vi "Test Manipulator API.vi"() -> ()   [LabVIEW 2020]
doc: "Manipulator API Tester."
uses:
  Settings/Named Position.ctl
  Manipulator.lvlib
panel:
  in  "Get Module Data":bool
  in  "Position Name":string
  out "Selected Target Position":string
  in  "Named Positions":i32(listbox)
  in  "Delete Named Position":bool
  in  "Add Named Position":bool
  in  "Move to Named Position":bool
  out "Axis Indicator":bool[](array[boolean])
  out "Speed (g)":dbl[](array[numeric])
  out "Pos (g)":dbl[](array[numeric])
  in  "Speed (s)":dbl[](array[numeric])
  in  "Pos (s)":dbl[](array[numeric])
  in  "Axis":i32
  in  "Move Axis with Speed":bool
  in  "Get Status":bool
  in  "Move Axis":bool
  in  "Get Position and Speed":bool
  out "Num Axes":i32
  in  "Get Num Axes":bool
  in  "Show Block Diagram":bool
  in  "Stop Module":bool
  in  "Start Module":bool
  in  "Hide Module Panel":bool
  in  "Show Module Panel":bool
  out "Status":string
  out "Module Running?":bool
  # "This VI tests the API for the Module."
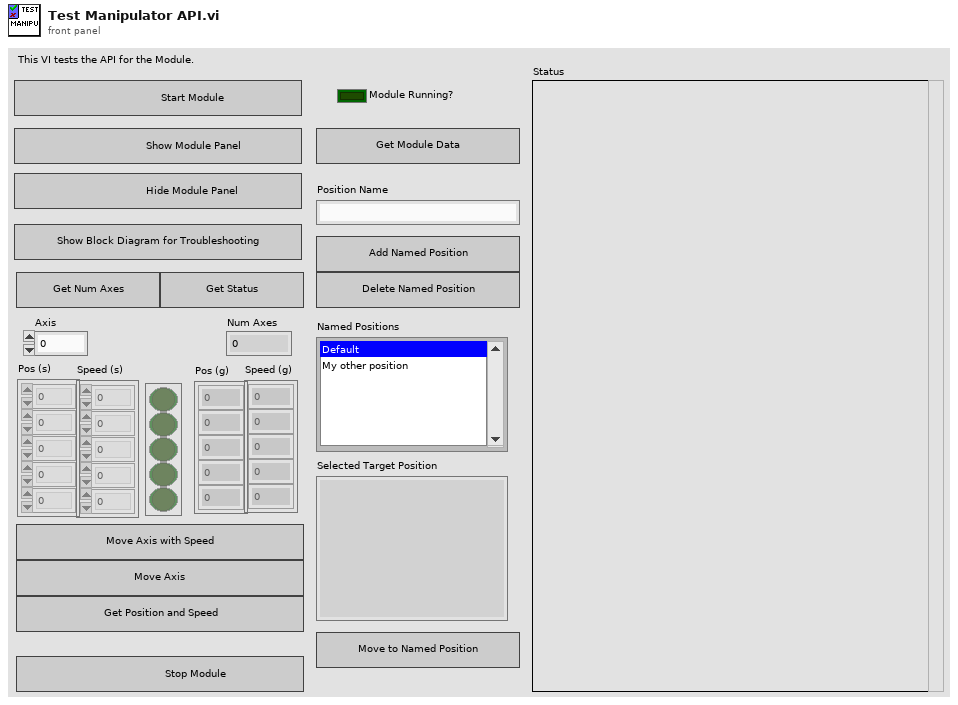
[diagram p1: front panel]
types:
  T1 = typedef "Manipulator.lvlib/Broadcast Events--cluster.ctl" = cluster{"Module Did Init":refnum<user-event>, "Status Updated":refnum<user-event>, "Error Reported":refnum<user-event>, "Module Did Stop":refnum<user-event>, "Update Module Execution Status":refnum<user-event>, "Broadcast Num Axes":refnum<user-event>, "Broadcast Position and Speed":refnum<user-event>, "Broadcast Status":refnum<user-event>}
  T2 = typedef "Manipulator.lvlib/Named Position.ctl" = cluster{"positions":dbl[], "name":string}
  T3 = typedef "Manipulator CLI Driver.lvlib/Manipulator Status.ctl" = enum16{"Moving", "Done", "Aborted", "Error", "No Status"}
  T4 = typedef "Manipulator.lvlib/Module Data--cluster.ctl" = cluster{"-Status":string, "_num_axes":i32, "positions":dbl[], "speeds":dbl[], "-named_positions":T2[]}
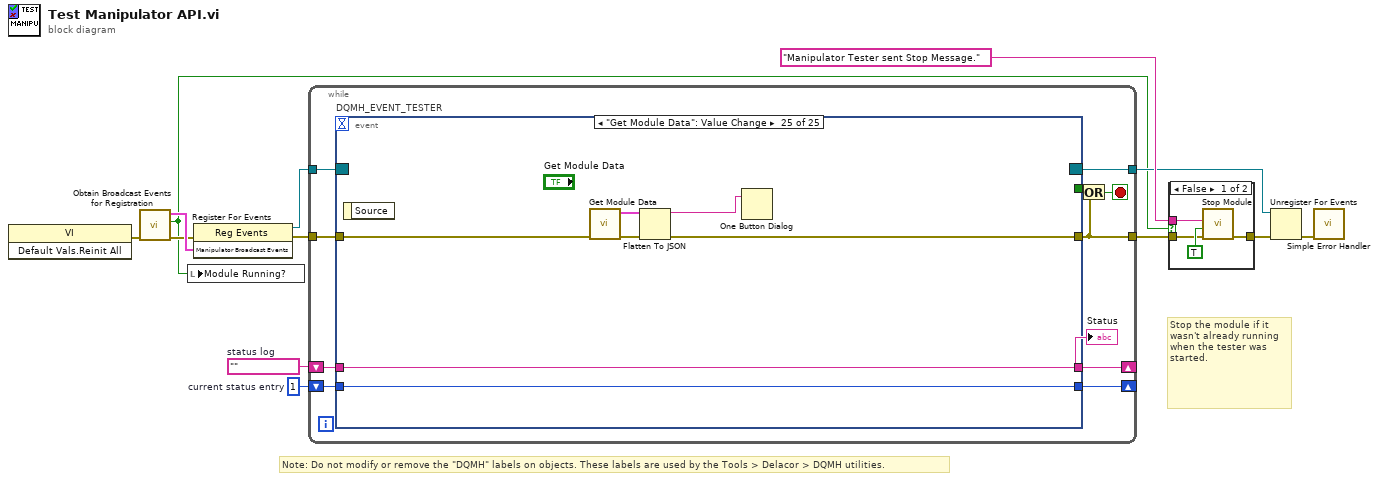
[diagram p0: block diagram]
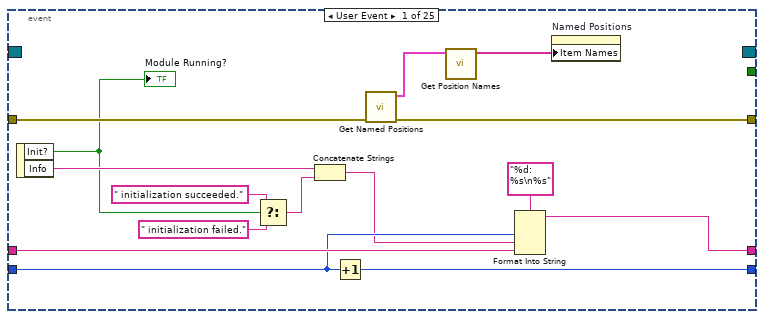
[diagram p3: hidden frame]
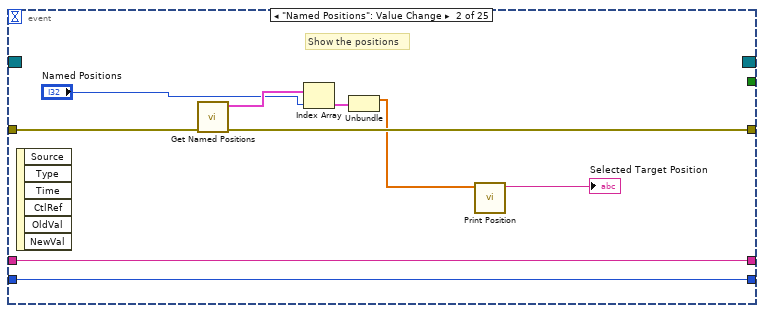
[diagram p4: hidden frame]
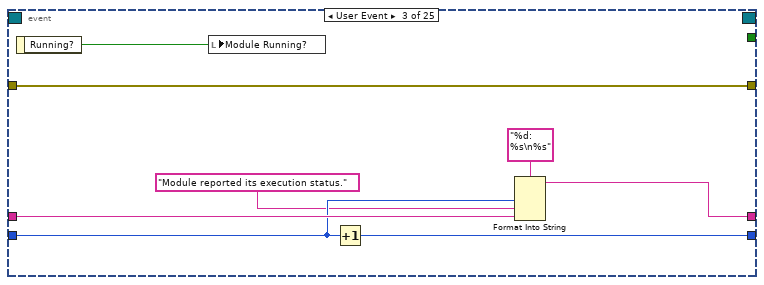
[diagram p5: hidden frame]
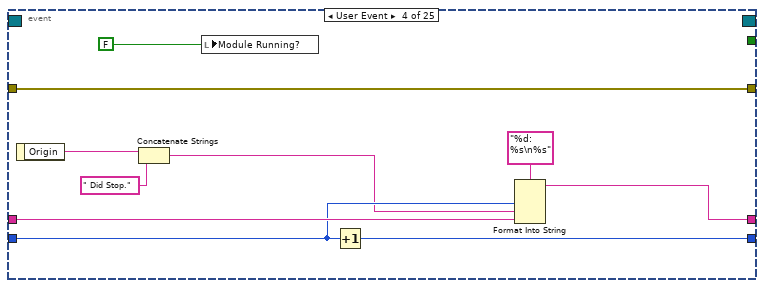
[diagram p6: hidden frame]
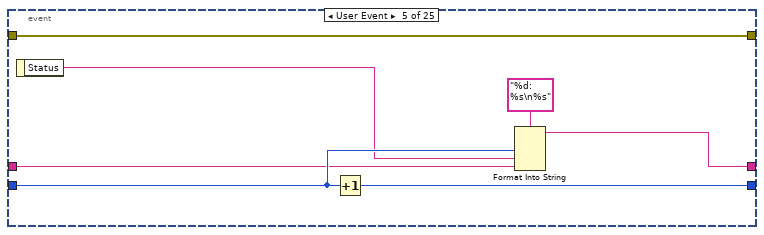
[diagram p7: hidden frame]
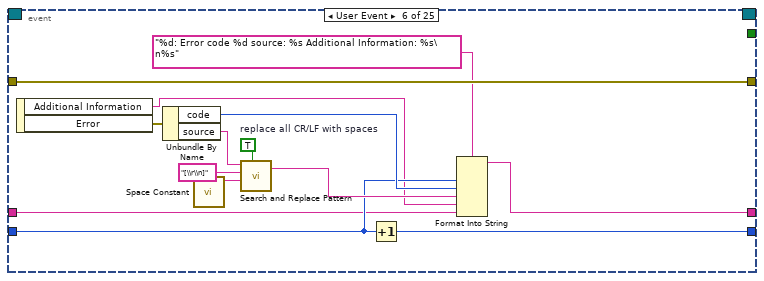
[diagram p8: hidden frame]
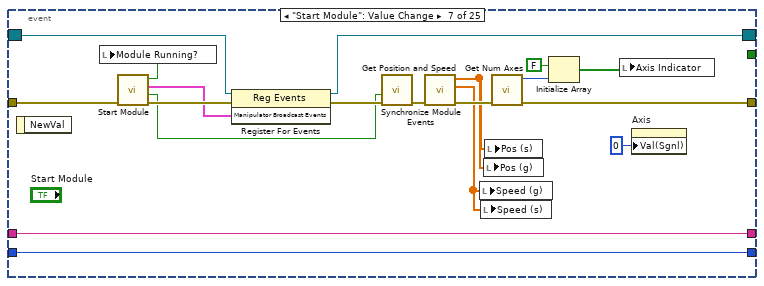
[diagram p9: hidden frame]
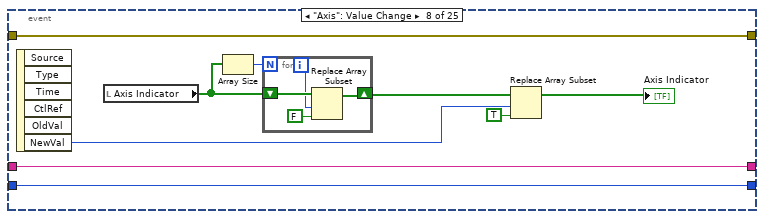
[diagram p10: hidden frame]
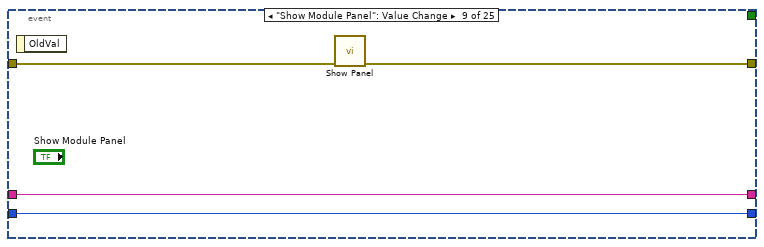
[diagram p11: hidden frame]
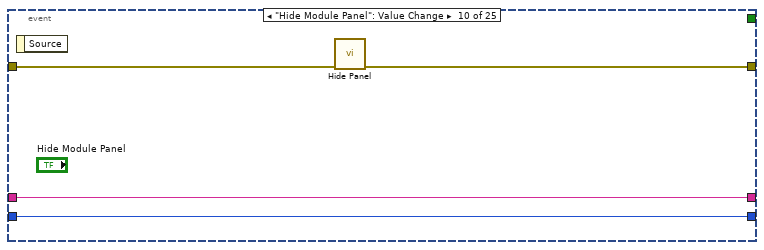
[diagram p12: hidden frame]
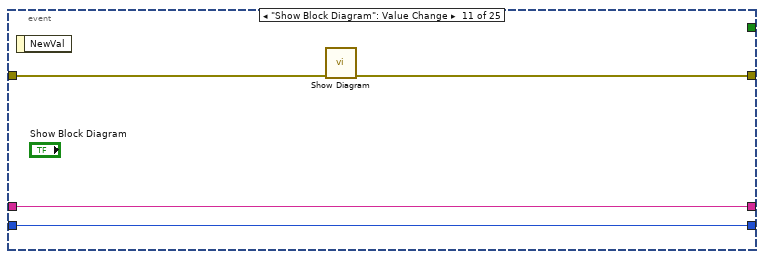
[diagram p13: hidden frame]
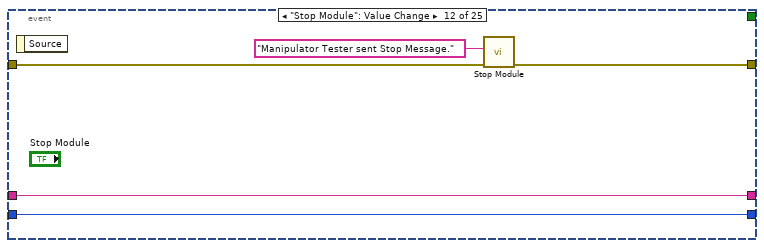
[diagram p14: hidden frame]
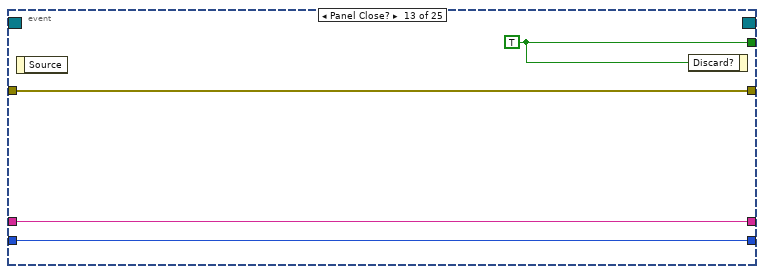
[diagram p15: hidden frame]
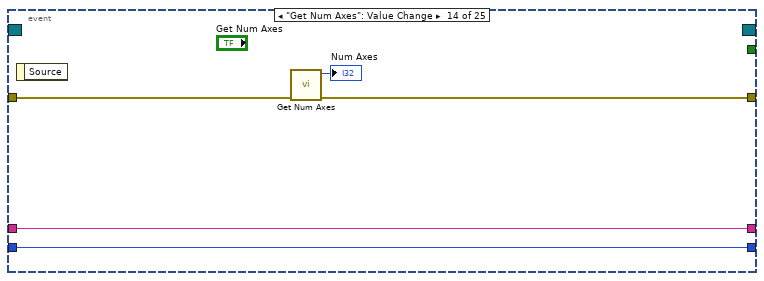
[diagram p16: hidden frame]
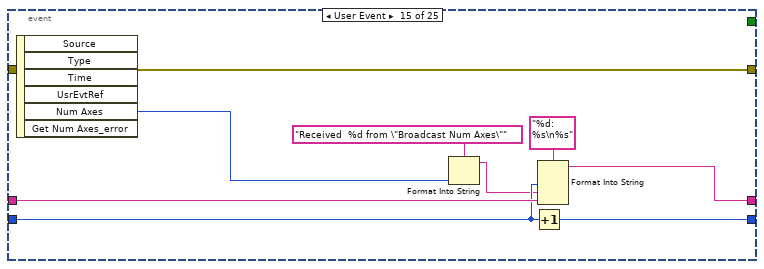
[diagram p17: hidden frame]
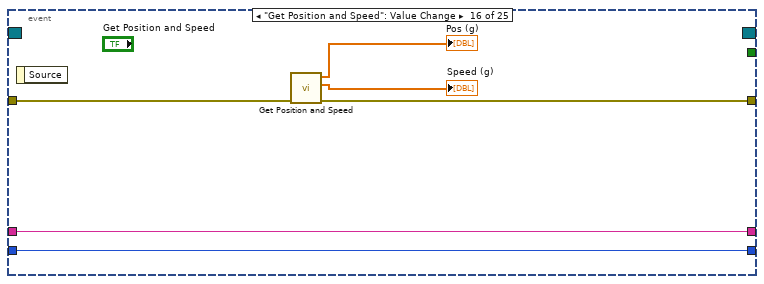
[diagram p18: hidden frame]
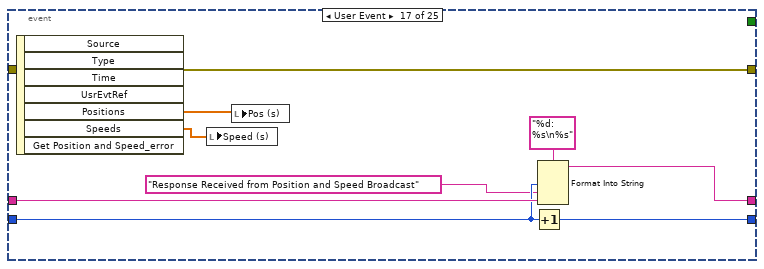
[diagram p19: hidden frame]
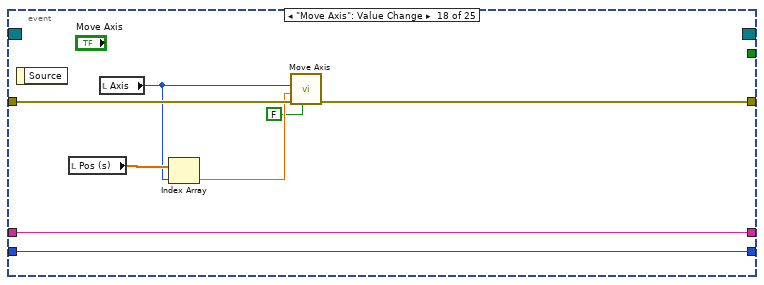
[diagram p20: hidden frame]
diagram:
  w10 = 1  # current status entry
  w11 = ""  # status log
  # "Stop the module if it wasn't already running when the tester was started."
  # "Note: Do not modify or remove the \"DQMH\" labels on objects. These labels are used by the Tools > Delacor > DQMH utilities."
  n1 = invoke class="VI" method="Default Vals.Reinit All"() -> (error out=w5:errorcluster)  [unwired: 3 in, 2 out]
  n2 = call "Obtain Broadcast Events for Registration.vi"("error in (no error)"=w5) -> ("error out"=w4:errorcluster, "Already running?"=w3:bool, "Manipulator Broadcast Events"=w8:T1)  [unwired: 8 in]
  n3 = local write "Module Running?"(w3) -> ()
  n4 = register-events(error in=w4, w8) -> (reference out=w7:refnum<event-registration>, error out=w9:errorcluster)  [unwired: 1 in]
  n5 = while {
    tunnel: w7 -> [w23]
    tunnel: [w14] -> w2
    shift-right: [w18] -> _
    shift-left: w11 -> [w20]
    shift-right: [w19] -> _
    shift-left: w10 -> [w21]
    tunnel: w9 -> [w16]
    tunnel: [w15] -> w6
    stop <- w17 stop-if-true
    n6 = event "DQMH_EVENT_TESTER" shown="[24] \"Get Module Data\": Value Change" {
      selector: w23 -> [_ _ _ _ _ _ w99 _ _ _ _ _ _ _ _ _ _ _ _ _ _ _ _ _ _]
      dyn-events: [_ _ _ _ _ _ w98 _ _ _ _ _ _ _ _ _ _ _ _ _ _ _ _ _ _] -> w15
      timeout: _ -> [_ _ _ _ _ _ _ _ _ _ _ _ _ _ _ _ _ _ _ _ _ _ _ _ _]
      tunnel: [_ _ _ _ _ _ _ _ _ _ _ _ w139 _ _ _ _ _ _ _ _ _ _ _ _] -> w22
      tunnel: [w26 w44 w49 w56 w66 w86 w91 w114 w122 w126 w127 w133 w136 w141 w153 w156 w168 w173 w177 w189 w196 w205 w215 w222 w228] -> w14
      tunnel: w21 -> [w35 w45 w53 w63 w69 w76 w102 w112 w120 w124 w128 w134 w137 w142 w150 w157 w165 w174 w178 w186 w197 w206 w216 w223 w230]
      tunnel: w20 -> [w36 w46 w54 w64 w68 w74 w103 w113 w121 w125 w129 w135 w138 w143 w152 w158 w167 w175 w179 w188 w198 w207 w217 w224 w231]
      tunnel: [w33 w46 w51 w61 w70 w77 w103 w113 w121 w125 w129 w135 w138 w143 w151 w158 w166 w175 w179 w187 w198 w207 w217 w224 w231] -> w18
      tunnel: [w34 w45 w52 w62 w72 w75 w102 w112 w120 w124 w128 w134 w137 w142 w149 w157 w164 w174 w178 w185 w197 w206 w216 w223 w230] -> w19
      tunnel: w16 -> [w38 w47 w49 w56 w66 w86 w96 w114 w119 w123 w130 w131 w136 w144 w153 w159 w168 w176 w180 w189 w199 w208 w218 w225 w232]
      event User Event {
        n7 = event-data() -> ("Init?"=w30:bool, "Info"=w32:string)  [unwired: 1 in]
        "Module Running?" <- w30
        n8 = Select(t=" initialization succeeded.", s=w30, f=" initialization failed.") -> (s? t:f=w27:string)
        n9 = Concatenate Strings(w32, w27) -> (w31:string)
        n10 = Increment(x=w35) -> (x+1=w34:i32)
        n11 = call "Get Named Positions.vi"("error in"=w38) -> ("error out"=w26:errorcluster, "Named Positions"=w25:T2[])  [unwired: 8 in, 1 out]
        n12 = call "Get Position Names.vi"("Named Positions"=w25) -> ("Array"=w24:string[])  [unwired: 10 in]
        n13 = Format Into String(format string="%d: %s\n%s", w35, w31, w36) -> (resulting string=w33:string)  [unwired: 2 in, 1 out]
        n14 = property on="Named Positions" class="LstBox (strict)"("Item Names"=w24) -> ()  [unwired: 2 in, 2 out]
      }
      event "Named Positions": Value Change {
        # "Show the positions"
        n15 = event-data() -> ()  [unwired: 1 in, 6 out]
        n16 = call "Get Named Positions.vi"("error in"=w47) -> ("error out"=w44:errorcluster, "Named Positions"=w43:T2[])  [unwired: 8 in, 1 out]
        n17 = Index Array(array=w43, index="Named Positions") -> (element=w41:T2)
        n18 = Unbundle(w41) -> ("positions"=w40:dbl[])  [unwired: 1 out]
        n19 = call "Print Position.vi"("positions"=w40) -> ("String"=→"Selected Target Position":string)  [unwired: 10 in]
      }
      event User Event {
        n20 = event-data() -> ("Running?"=w48:bool)  [unwired: 1 in]
        n21 = local write "Module Running?"(w48) -> ()
        n22 = Increment(x=w53) -> (x+1=w52:i32)
        n23 = Format Into String(format string="%d: %s\n%s", w53, "Module reported its execution status.", w54) -> (resulting string=w51:string)  [unwired: 2 in, 1 out]
      }
      event User Event {
        n24 = event-data() -> ("Origin"=w60:string)  [unwired: 1 in]
        n25 = Concatenate Strings(w60, " Did Stop.") -> (w59:string)
        n26 = local write "Module Running?"(FALSE ("Module Did Init?")) -> ()
        n27 = Increment(x=w63) -> (x+1=w62:i32)
        n28 = Format Into String(format string="%d: %s\n%s", w63, w59, w64) -> (resulting string=w61:string)  [unwired: 2 in, 1 out]
      }
      event User Event {
        n29 = event-data() -> ("Status"=w67:string)  [unwired: 1 in]
        n30 = Increment(x=w69) -> (x+1=w72:i32)
        n31 = Format Into String(format string="%d: %s\n%s", w69, w67, w68) -> (resulting string=w70:string)  [unwired: 2 in, 1 out]
      }
      event User Event {
        w82 = TRUE  # replace all CR/LF with spaces
        n32 = event-data() -> ("Additional Information"=w73:string, "Error"=w78:errorcluster)  [unwired: 1 in]
        n33 = Unbundle By Name(w78) -> ("code"=w79:i32, "source"=w80:string)
        n34 = call <vilib>:"Space Constant.vi"() -> ("String"=w83:string)
        n35 = call <vilib>:"Search and Replace Pattern.vi"("string"=w80, "regular expression (\"\")"="[\\r\\n]" ("regular expression (\"\")"), "replace string (\"\")"=w83, "replace all? (F)"=w82) -> ("result string"=w81:string)  [unwired: 1 in, 1 out]
        n36 = Increment(x=w76) -> (x+1=w75:i32)
        n37 = Format Into String(format string="%d: Error code %d source: %s Additional Information: %s\n%s", w76, w79, w81, w73, w74) -> (resulting string=w77:string)  [unwired: 2 in, 1 out]
      }
      event "Start Module": Value Change {
        n38 = event-data() -> ()  [unwired: 1 in, 1 out]
        n39 = call "Start Module.vi"("error in (no error)"=w96) -> ("error out"=w104:errorcluster, "Wait for Event Sync?"=w101:bool, "Manipulator Broadcast Events"=w100:T1, "Module Was Already Running?"=w95:bool)  [unwired: 7 in]
        n40 = local write "Module Running?"(w95) -> ()
        n41 = register-events(reference=w99, error in=w104, w100) -> (reference out=w98:refnum<event-registration>, error out=w105:errorcluster)
        n42 = call "Synchronize Module Events.vi"("error in"=w105, "Wait for Event Sync?"=w101) -> ("error out"=w97:errorcluster)  [unwired: 9 in]
        n43 = call "Get Position and Speed.vi"("error in"=w97) -> ("error out"=w94:errorcluster, "Speeds"=w93:dbl[], "Positions"=w92:dbl[])  [unwired: 7 in, 1 out]
        n44 = local write "Speed (g)"(w93) -> ()
        n45 = local write "Speed (s)"(w93) -> ()
        n46 = local write "Pos (g)"(w92) -> ()
        n47 = local write "Pos (s)"(w92) -> ()
        n48 = call "Get Num Axes.vi"("error in"=w94) -> ("error out"=w91:errorcluster, "Num Axes"=w88:i32)  [unwired: 8 in, 1 out]
        n49 = Initialize Array(FALSE, w88) -> (w89:bool[])
        n50 = local write "Axis Indicator"(w89) -> ()
        n51 = property on="Axis" class="DigNum (strict)"("Val(Sgnl)"=0 ("Value (Signaling)")) -> ()  [unwired: 2 in, 2 out]
      }
      event "Axis": Value Change {
        n52 = event-data() -> ("NewVal"=w109:i32)  [unwired: 1 in, 5 out]
        n53 = local read "Axis Indicator"() -> (w106:bool[])
        n54 = Array Size(array=w106) -> (size(s)=w107:i32)
        n55 = for {
          N: w107 -> [_]
          shift-right: [w116] -> w111
          shift-left: w106 -> [w118]
          i -> [w115]
          n56 = Replace Array Subset(array=w118, new element=FALSE ("new element/subarray"), index=w115) -> (w116:bool[])
        }
        n57 = Replace Array Subset(array=w111, new element=TRUE ("new element/subarray"), index=w109) -> (→"Axis Indicator":bool[])
      }
      event "Show Module Panel": Value Change {
        n58 = event-data() -> ()  [unwired: 1 in, 1 out]
        n59 = call "Show Panel.vi"("error in (no error)"=w119) -> ("error out"=w122:errorcluster)  [unwired: 10 in]
      }
      event "Hide Module Panel": Value Change {
        n60 = event-data() -> ()  [unwired: 1 in, 1 out]
        n61 = call "Hide Panel.vi"("error in (no error)"=w123) -> ("error out"=w126:errorcluster)  [unwired: 10 in]
      }
      event "Show Block Diagram": Value Change {
        n62 = event-data() -> ()  [unwired: 1 in, 1 out]
        n63 = call "Show Diagram.vi"("error in (no error)"=w130) -> ("error out"=w127:errorcluster)  [unwired: 10 in]
      }
      event "Stop Module": Value Change {
        n64 = event-data() -> ()  [unwired: 1 in, 1 out]
        n65 = call "Stop Module.vi"("error in"=w131, "Origin"="Manipulator Tester sent Stop Message.") -> ("error out"=w133:errorcluster)  [unwired: 9 in]
      }
      event Panel Close? {
        w139 = TRUE ("Discard?")
        n66 = event-data() -> ()  [unwired: 1 in, 1 out]
        n67 = event-data("Discard?"=w139) -> ()  [unwired: 1 in, 1 out]
      }
      event "Get Num Axes": Value Change {
        n68 = event-data() -> ()  [unwired: 1 in, 1 out]
        n69 = call "Get Num Axes.vi"("error in"=w144) -> ("error out"=w141:errorcluster, "Num Axes"=→"Num Axes":i32)  [unwired: 8 in, 1 out]
      }
      event User Event {
        n70 = event-data() -> ("Num Axes"=w145:i32)  [unwired: 1 in, 5 out]
        n71 = Format Into String(format string="Received  %d from \"Broadcast Num Axes\"", w145) -> (resulting string=w146:string)  [unwired: 2 in, 1 out]
        n72 = Increment(x=w150) -> (x+1=w149:i32)
        n73 = Format Into String(format string="%d: %s\n%s", w150, w146, w152) -> (resulting string=w151:string)  [unwired: 2 in, 1 out]
      }
      event "Get Position and Speed": Value Change {
        n74 = event-data() -> ()  [unwired: 1 in, 1 out]
        n75 = call "Get Position and Speed.vi"("error in"=w159) -> ("error out"=w156:errorcluster, "Speeds"=→"Speed (g)":dbl[], "Positions"=→"Pos (g)":dbl[])  [unwired: 7 in, 1 out]
      }
      event User Event {
        n76 = event-data() -> ("Positions"=w161:dbl[], "Speeds"=w160:dbl[])  [unwired: 1 in, 5 out]
        n77 = local write "Speed (s)"(w160) -> ()
        n78 = local write "Pos (s)"(w161) -> ()
        n79 = Increment(x=w165) -> (x+1=w164:i32)
        n80 = Format Into String(format string="%d: %s\n%s", w165, "Response Received from Position and Speed Broadcast" ("format string"), w167) -> (resulting string=w166:string)  [unwired: 2 in, 1 out]
      }
      event "Move Axis": Value Change {
        n81 = event-data() -> ()  [unwired: 1 in, 1 out]
        n82 = local read "Pos (s)"() -> (w172:dbl[])
        n83 = local read "Axis"() -> (w170:i32)
        n84 = Index Array(array=w172, index=w170) -> (element=w171:dbl)
        n85 = call "Move Axis.vi"("wait for reply (T)"=FALSE, "error in"=w176, "Position"=w171, "Axis"=w170) -> ("error out"=w173:errorcluster)  [unwired: 6 in, 1 out]
      }
      event "Get Status": Value Change {
        n86 = event-data() -> ()  [unwired: 1 in, 1 out]
        n87 = call "Get Status.vi"("error in"=w180) -> ("error out"=w177:errorcluster)  [unwired: 8 in, 2 out]
      }
      event User Event {
        n88 = event-data() -> ("Status"=w181:T3)  [unwired: 1 in, 5 out]
        n89 = Format Into String(format string="Broadcasted Status - %s", w181) -> (resulting string=w182:string)  [unwired: 2 in, 1 out]
        n90 = Increment(x=w186) -> (x+1=w185:i32)
        n91 = Format Into String(format string="%d: %s\n%s", w186, w182, w188) -> (resulting string=w187:string)  [unwired: 2 in, 1 out]
      }
      event "Move Axis with Speed": Value Change {
        n92 = event-data() -> ()  [unwired: 1 in, 1 out]
        n93 = Index Array(array="Speed (s)", index="Axis") -> (element=w194:dbl)
        n94 = Index Array(array="Pos (s)", index="Axis") -> (element=w191:dbl)
        n95 = call "Move Axis with Speed.vi"("wait for reply (T)"=FALSE, "Axis"="Axis", "error in"=w199, "Speed"=w194, "Position"=w191) -> ("error out"=w196:errorcluster)  [unwired: 5 in, 1 out]
      }
      event "Move to Named Position": Value Change {
        # "don't wait for reply.\nthis would take too long"
        n96 = event-data() -> ()  [unwired: 1 in, 1 out]
        n97 = local read "Named Positions"() -> (w202:i32)
        n98 = call "Get Named Positions.vi"("error in"=w208) -> ("error out"=w204:errorcluster, "Named Positions"=w203:T2[])  [unwired: 8 in, 1 out]
        n99 = Index Array(array=w203, index=w202) -> (element=w201:T2)
        n100 = call "Move to Named Position.vi"("wait for reply (T)"=FALSE, "error in"=w204, "named_position"=w201) -> ("error out"=w205:errorcluster)  [unwired: 7 in, 1 out]
      }
      event "Add Named Position": Value Change {
        n101 = event-data() -> ()  [unwired: 1 in, 1 out]
        n102 = local read "Pos (s)"() -> (w212:dbl[])
        n103 = Bundle By Name(cluster=T2 {"positions"=[], "name"=""} ("named_position"), "positions"=w212, "name"="Position Name") -> (w211:T2)
        n104 = call "Add Named Position.vi"("error in"=w218, "Named Position"=w211) -> ("error out"=w215:errorcluster, "Named Positions"=w210:T2[])  [unwired: 7 in, 1 out]
        n105 = call "Get Position Names.vi"("Named Positions"=w210) -> ("Array"=w209:string[])  [unwired: 10 in]
        n106 = property on="Named Positions" class="LstBox (strict)"("Item Names"=w209) -> ()  [unwired: 2 in, 2 out]
      }
      event "Delete Named Position": Value Change {
        n107 = event-data() -> ()  [unwired: 1 in, 1 out]
        n108 = local read "Named Positions"() -> (w221:i32)
        n109 = call "Delete Named Position.vi"("error in"=w225, "Index"=w221) -> ("error out"=w222:errorcluster, "Named Positions"=w220:T2[])  [unwired: 7 in, 1 out]
        n110 = call "Get Position Names.vi"("Named Positions"=w220) -> ("Array"=w219:string[])  [unwired: 10 in]
        n111 = property on="Named Positions" class="LstBox (strict)"("Item Names"=w219) -> ()  [unwired: 2 in, 2 out]
      }
      event "Get Module Data": Value Change {
        n112 = event-data() -> ()  [unwired: 1 in, 1 out]
        n113 = call "Get Module Data.vi"("error in"=w232) -> ("error out"=w229:errorcluster, "Module Data"=w227:T4)  [unwired: 8 in, 1 out]
        n114 = Flatten To JSON(anything=w227, error in (no error)=w229) -> (JSON string=w226:string, 11:w228:errorcluster)  [unwired: 1 in]
        n115 = One Button Dialog(message=w226) -> ()  [unwired: 1 in, 1 out]
      }
    }
    "Status" <- w18
    n116 = Or(x=w22, y=w14) -> (x .or. y?=w17:bool)
  }
  n117 = case shown="False" w3 {
    tunnel: [w236 w237] -> w13
    tunnel: "Manipulator Tester sent Stop Message." ("Origin") -> [w235 _]
    tunnel: w2 -> [w233 w237]
    frame False {
      n118 = call "Stop Module.vi"("error in"=w233, "Wait for Module to Stop? (F)"=TRUE ("Wait for Module to stop?"), "Origin"=w235) -> ("error out"=w236:errorcluster)  [unwired: 8 in]
    }
    frame True {
    }
  }
  n119 = Unregister For Events(event registration refnum=w6, error in=w13) -> (error out=w1:errorcluster)
  n120 = call <vilib>:"Simple Error Handler.vi"("error in (no error)"=w1) -> ()  [unwired: 4 in, 5 out]
